vi "transformedProductColumnInformation.vi"(8 "error in":errorcluster, 11 "columnInformationReading":T2(array[cluster])) -> (0 "error out":errorcluster, 3 "columnInformationReadingTransformed":string[](array[string]))   [LabVIEW 2014]
uses:
  <vilib>/addons/database/Auxilliary.llb/DB Tools DataTypes.ctl
  <vilib>/addons/database/NI_Database_API.lvlib
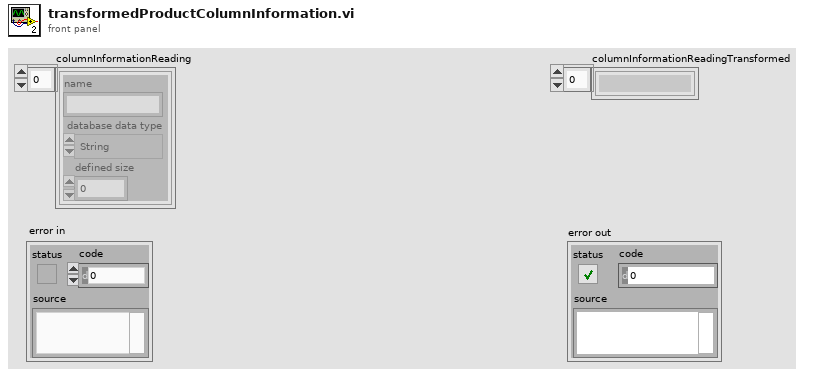
[diagram p1: front panel]
types:
  T1 = typedef "NI_Database_API.lvlib/DB Tools DataTypes.ctl" = enum16{"String", "Long (I32)", "Single (SGL)", "Double (DBL)", "Date/Time", "Binary"}
  T2 = cluster{"name":string, "database data type":T1, "defined size":i32}[]
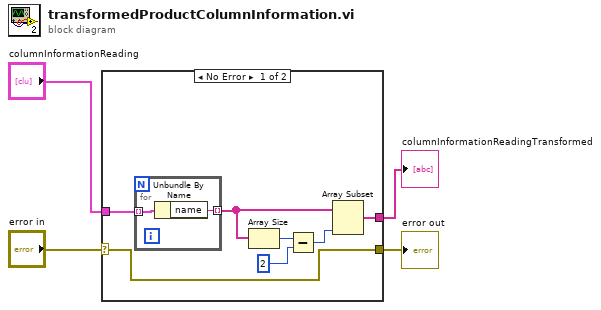
[diagram p0: block diagram]
diagram:
  n1 = case shown="No Error" "error in" {
    selector: "error in" -> [w5 w14]
    tunnel: "columnInformationReading" -> [w11 _]
    tunnel: [w10 _] -> w3
    tunnel: [w5 w14] -> w1
    frame No Error {
      n2 = for {
        tunnel: w11 -> [w12] mode=indexing
        tunnel: [w13] -> w6 mode=indexing
        n3 = Unbundle By Name(w12) -> ("name"=w13:string)
      }
      n4 = Array Size(array=w6) -> (size(s)=w9:i32)
      n5 = Subtract(x=w9, y=2) -> (x-y=w8:i32)
      n6 = Array Subset(array=w6, length=w8) -> (w10:string[])  [unwired: 1 in]
    }
    frame Error {
    }
  }
  "columnInformationReadingTransformed" <- w3
  "error out" <- w1
